vi "File Manager.vi"(7 "Operation (0: Create Directory)":u16(ring) items=["Create Directory", "Copy File", "Delete Directory"], 8 "error in (no error)":errorcluster, 9 "Destination ()":string, 10 "Source ()":string, 11 "VISA resource name":refnum<visa-resource-name>) -> (0 "error out":errorcluster, 3 "VISA resource name out":refnum<visa-resource-name>)   [LabVIEW 2022 SP3, in "Agilent ENA Series.lvlib"]
doc: "Creates, deletes directory or copies a file."
uses:
  <instrlib>/Agilent ENA Series/Agilent ENA Series.lvlib
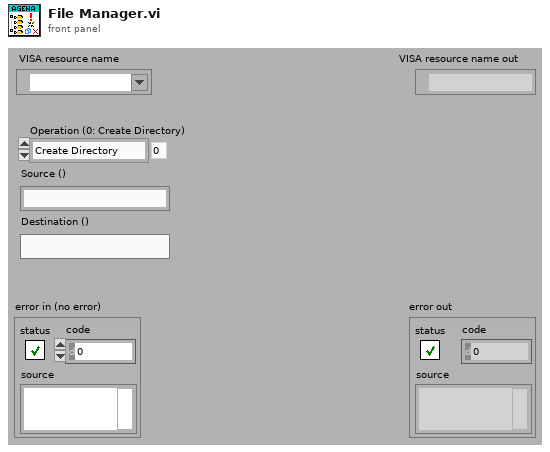
[diagram p1: front panel]
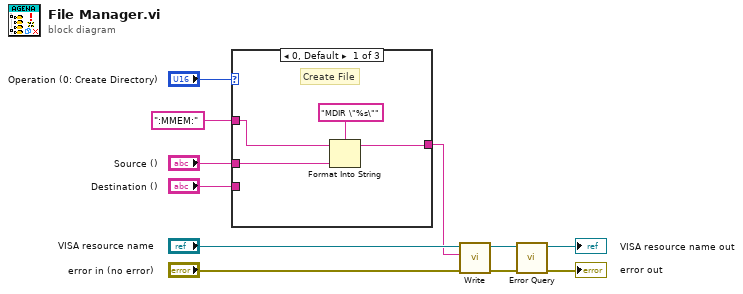
[diagram p0: block diagram]
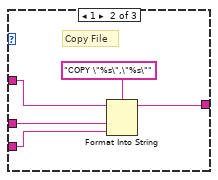
[diagram p2: hidden frame]
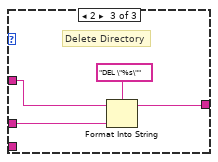
[diagram p3: hidden frame]
diagram:
  n1 = case shown="0, Default" "Operation (0: Create Directory)" {
    tunnel: "Source ()" -> [w14 w19 w23]
    tunnel: "Destination ()" -> [_ w18 _]
    tunnel: [w13 w17 w22] -> w6
    tunnel: ":MMEM:" -> [w12 w16 w21]
    frame 0, Default {
      # "Create File"
      n2 = Format Into String(format string="MDIR \"%s\"", initial string=w12, w14) -> (resulting string=w13:string)  [unwired: 1 in, 1 out]
    }
    frame 1 {
      # "Copy File"
      n3 = Format Into String(format string="COPY \"%s\",\"%s\"", initial string=w16, w19, w18) -> (resulting string=w17:string)  [unwired: 1 in, 1 out]
    }
    frame 2 {
      # "Delete Directory"
      n4 = Format Into String(format string="DEL \"%s\"", initial string=w21, w23) -> (resulting string=w22:string)  [unwired: 1 in, 1 out]
    }
  }
  n5 = call <instrlib>:"Write.vi"("error in (no error)"="error in (no error)", "String ()"=w6, "VISA resource name"="VISA resource name") -> ("error out"=w3:errorcluster, "VISA resource name out"=w4:refnum<visa-resource-name>)  [unwired: 6 in, 1 out]
  n6 = call <instrlib>:"Error Query.vi"("error in (no error)"=w3, "VISA resource name"=w4) -> ("error out"=→"error out":errorcluster, "VISA resource name out"=→"VISA resource name out":refnum<visa-resource-name>)  [unwired: 6 in, 2 out]
